vi "Set BackColor.vi"(8 "error in (no error)":errorcluster, 10 "Color.lvclass":refnum<class "Color.lvclass">, 11 "View in":refnum<class "Cell View.lvclass">) -> (0 "error out":errorcluster, 3 "View out":refnum<class "Cell View.lvclass">)   [LabVIEW 2024, in "Cell View.lvclass"]
uses:
  Cell View.lvclass
  Color/Color.lvclass
  Cell View.lvclass/Cell View.ctl
  Color/Color.lvclass/Color.ctl
  D:/git/Sourcegrid-LabVIEW/dll/SourceGrid.dll
  dll/SourceGrid.dll
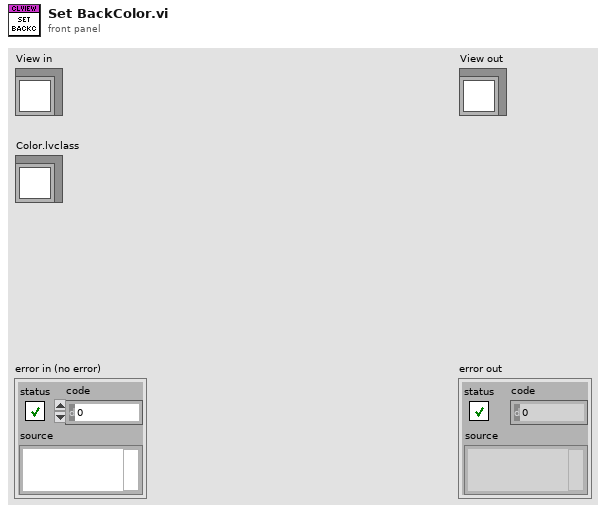
[diagram p1: front panel]
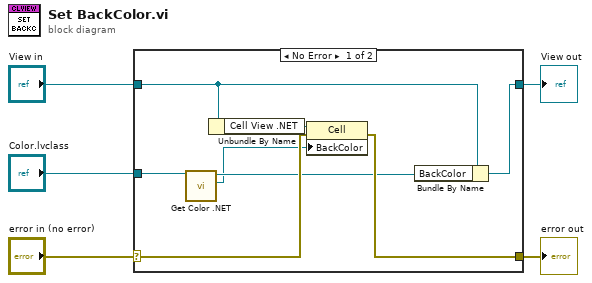
[diagram p0: block diagram]
diagram:
  n1 = case shown="No Error" "error in (no error)" {
    selector: "error in (no error)" -> [w10 w14]
    tunnel: [w9 w14] -> w4
    tunnel: [w13 w15] -> w2
    tunnel: "View in" -> [w12 w15]
    tunnel: "Color.lvclass" -> [w8 _]
    frame No Error {
      n2 = call "Get Color .NET.vi"("Color in"=w8) -> ("Color .NET"=w6:refnum<k24>, "Color out"=w7:refnum<class "Color.lvclass">)  [unwired: 9 in]
      n3 = Unbundle By Name(w12) -> ("Cell View .NET"=w11:refnum<k24>)
      n4 = property class="Cell"(reference=w11, error in=w10, "BackColor"=w6) -> (error out=w9:errorcluster)  [unwired: 1 out]
      n5 = Bundle By Name(cluster=w12, "BackColor"=w7) -> (w13:refnum<class "Cell View.lvclass">)
    }
    frame Error {
    }
  }
  "error out" <- w4
  "View out" <- w2
